vi "generate key value pairs.vi"(11 "key-value pairs":cluster{"key":string, "value":string}[](array[cluster])) -> (3 "stream":string)   [LabVIEW 2013]
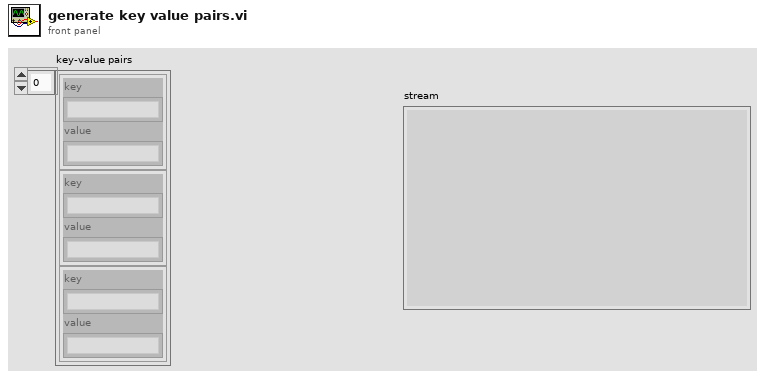
[diagram p1: front panel]
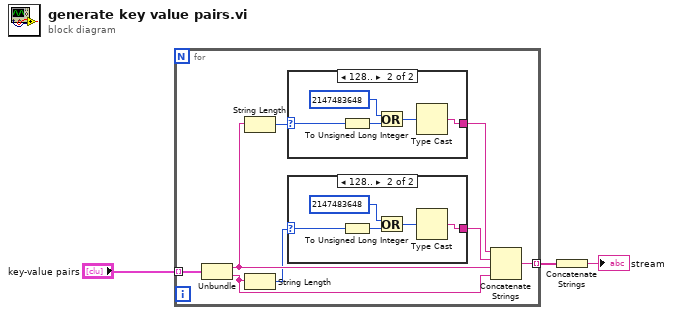
[diagram p0: block diagram]
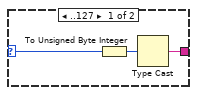
[diagram p2: hidden frame]
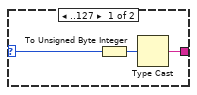
[diagram p3: hidden frame]
diagram:
  n1 = for {
    tunnel: "key-value pairs" -> [w11] mode=indexing
    tunnel: [w9] -> w2 mode=indexing
    n2 = Unbundle(w11) -> ("key"=w7:string, "value"=w4:string)
    n3 = String Length(string=w7) -> (length=w10:i32)
    n4 = String Length(string=w4) -> (length=w6:i32)
    n5 = case shown="128.." w10 {
      selector: w10 -> [w22 w27]
      tunnel: [w20 w23] -> w8
      frame ..127 {
        n6 = To Unsigned Byte Integer(number=w22) -> (unsigned 8bit integer=w21:u8)
        n7 = Type Cast(x=w21) -> (*(type *) &x=w20:string)  [unwired: 1 in]
      }
      frame 128.. {
        n8 = To Unsigned Long Integer(number=w27) -> (unsigned 32bit integer=w26:u32)
        n9 = Or(x=u32 2147483648, y=w26) -> (x .or. y?=w24:u32)
        n10 = Type Cast(x=w24) -> (*(type *) &x=w23:string)  [unwired: 1 in]
      }
    }
    n11 = case shown="128.." w6 {
      selector: w6 -> [w14 w19]
      tunnel: [w12 w15] -> w5
      frame ..127 {
        n12 = To Unsigned Byte Integer(number=w14) -> (unsigned 8bit integer=w13:u8)
        n13 = Type Cast(x=w13) -> (*(type *) &x=w12:string)  [unwired: 1 in]
      }
      frame 128.. {
        n14 = To Unsigned Long Integer(number=w19) -> (unsigned 32bit integer=w18:u32)
        n15 = Or(x=u32 2147483648, y=w18) -> (x .or. y?=w16:u32)
        n16 = Type Cast(x=w16) -> (*(type *) &x=w15:string)  [unwired: 1 in]
      }
    }
    n17 = Concatenate Strings(w8, w5, w7, w4) -> (w9:string)
  }
  n18 = Concatenate Strings(w2) -> (→"stream":string)
